vi "SailSetSuggestions.vi"() -> ()   [LabVIEW 2012]
panel:
  in  "DesiredHeading":dbl
  in  "RobotHeading":dbl
  in  "RudderForce":dbl
  in  "DegreeOfLuffing":dbl
  in  "RelativeWindAngle":dbl
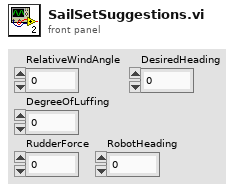
[diagram p1: front panel]
types:
  T1 = enum16{"Straight", "Turning", "Tacking", "Approach Maneuver", "Cross Wind (Tack)", "Cross Wind (Gybe)", "Turtle Mode", ""}
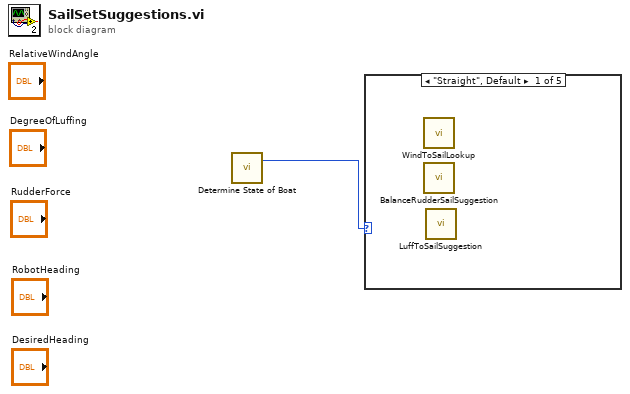
[diagram p0: block diagram]
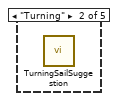
[diagram p2: hidden frame]
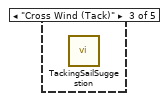
[diagram p3: hidden frame]
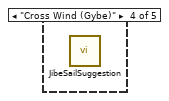
[diagram p4: hidden frame]
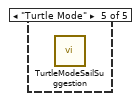
[diagram p5: hidden frame]
diagram:
  n1 = call "Determine State of Boat.vi"() -> ("State of Boat"=w1:T1)  [unwired: 11 in]
  n2 = case shown="\"Straight\", Default" w1 {
    frame "Straight", Default {
      n3 = call "WindToSailLookup.vi"() -> ()  [unwired: 12 in]
      n4 = call "BalanceRudderSailSuggestion.vi"() -> ()  [unwired: 12 in]
      n5 = call "LuffToSailSuggestion.vi"() -> ()  [unwired: 12 in]
    }
    frame "Turning" {
      n6 = call "TurningSailSuggestion.vi"() -> ()  [unwired: 12 in]
    }
    frame "Cross Wind (Tack)" {
      n7 = call "TackingSailSuggestion.vi"() -> ()  [unwired: 12 in]
    }
    frame "Cross Wind (Gybe)" {
      n8 = call "JibeSailSuggestion.vi"() -> ()  [unwired: 12 in]
    }
    frame "Turtle Mode" {
      n9 = call "TurtleModeSailSuggestion.vi"() -> ()  [unwired: 12 in]
    }
  }
